vi "serial-write.vi"(0 "VISA Name":refnum<visa-resource-name>="COM4", 1 "String to write":string="*IDN?\n") -> ()   [LabVIEW 2022 SP3]
doc: "The Basic Serial Write and Read (2Port) example opens 2 VISA resources and configures one COM port to perform a write operation and the other COM port to perform a read operation. This VI will wait until the specified number of bytes (bytes to read) is received at the port or until a termination character is read.\n\nINSTRUCTIONS:\n1) Select the serial resource and configuration parameters (baud rate, data bits, parity, stop bits, flow control).\n2) Select the operations to be performed. \n3) Connect a null modem RS-232 or RS-485/422 cable between the 2 ports.\n4) Run the VI to see the \"read string\" match the \"string to write\".\n\nLike the Basic Serial Write and Read VI, this VI allows you perform diagnostic tests on your ports. You can use this VI to perform a wrapback test. Both serial ports must have the same basic configuration parameters. You can connect two of the ports using a null modem cable, which effectively connects one port's RX lines to the other port's TX lines. If you use a straight-through cable, one port's RX lines will be connected to the other port's RX lines, and you cannot communicate between the two ports. \n\nOn the block diagram, the VI calls the VISA Configure Serial Port VI twice, once for each of the two ports. This opens two separate VISA sessions. One VISA session performs the Write operation and the other performs the Read operation. Because two VISA sessions are opened, the VI includes two separate VISA Close functions."
uses:
  <vilib>/Instr/_visa.llb/VISA Configure Serial Port (Instr).vi
panel:
  in  "Stop bits":u16(ring)=10 items=["1.0"=10, "1.5"=15, "2.0"=20]
  in  "Flow control":u16(ring) items=["None"=0, "XON/XOFF"=1, "RTS/CTS"=2, "DTR/DSR"=4]
  in  "Parity (0:none)":u16(ring) items=["None", "Odd", "Even", "Mark", "Space"]
  in  "Data bits (8)":u16=8 min=5 max=8 step=1
  in  "Baud Rate (9600)":u32=9600
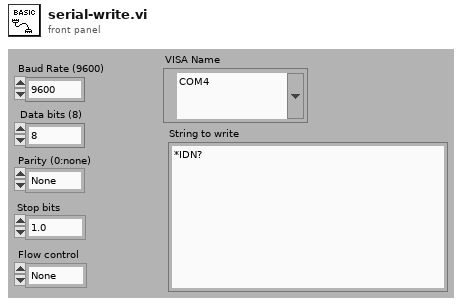
[diagram p1: front panel]
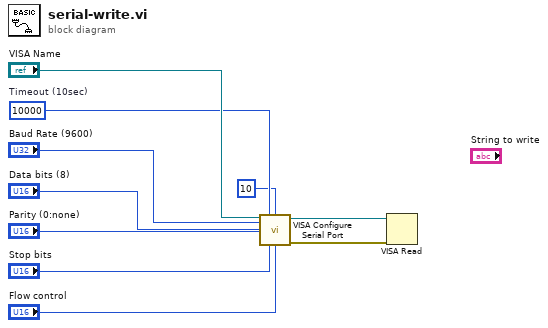
[diagram p0: block diagram]
diagram:
  w8 = u32 10000  # Timeout (10sec)
  n1 = call-poly "VISA Configure Serial Port"("VISA resource name"="VISA Name", "timeout (10sec)"=w8, "termination char\n(0xA = '\\n' = LF)"=u8 10 ("termination char\n(0xA = '\\n' = LF)"), "baud rate (9600)"="Baud Rate (9600)", "data bits (8)"="Data bits (8)", "parity (0:none)"="Parity (0:none)", "stop bits (10: 1 bit)"="Stop bits", "flow control (0:none)"="Flow control") -> ("VISA resource name out"=w9:refnum<visa-resource-name>, "error out"=w2:errorcluster)  [unwired: 2 in, 4 out]
  n2 = VISA Read(VISA resource name=w9, error in (no error)=w2) -> ()  [unwired: 1 in, 4 out]
